vi "ROI entry screen-sanity check fitting.vi"(5 "Array in":dbl[](array[numeric])) -> (1 "Equal to the first value?":bool[](array[boolean]), 2 "Array out":dbl[](array[numeric]))   [LabVIEW 2017]
panel:
  # "The first element is always FALSE"
  # "RE-ENTRANT"
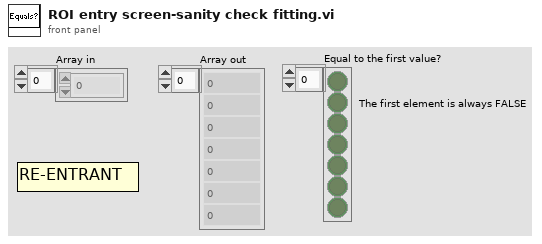
[diagram p1: front panel]
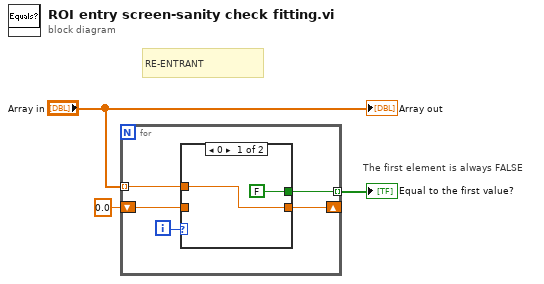
[diagram p0: block diagram]
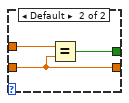
[diagram p2: hidden frame]
diagram:
  # "The first element is always FALSE"
  # "RE-ENTRANT"
  n1 = for {
    tunnel: "Array in" -> [w6] mode=indexing
    shift-right: [w7] -> _
    shift-left: 0.0 -> [w5]
    tunnel: [w4] -> w1 mode=indexing
    i -> [w8]
    n2 = case shown="0" w8 {
      tunnel: [w10 w12] -> w7
      tunnel: w6 -> [w10 w13]
      tunnel: w5 -> [_ w12]
      tunnel: [FALSE w11] -> w4
      frame 0 {
      }
      frame Default {
        n3 = Equal?(x=w13, y=w12) -> (x = y?=w11:bool)
      }
    }
  }
  "Equal to the first value?" <- w1
  "Array out" <- "Array in"
